vi "Abort.vi"() -> ()   [LabVIEW 2024]
uses:
  states.ctl
  <vilib>/regexp/Match Regular Expression.xnode
panel:
  out "RunningVIs":string[][](table)
  in  "Exit":bool
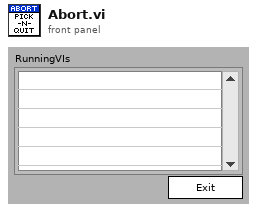
[diagram p1: front panel]
types:
  T1 = typedef "states.ctl" = enum16{"Idle", "Data: Initialize", "Data: get contexts", "Data: get running VIs", "Data: count running", "Macro: Initialize", "Macro: get VIs", "Script: abort VI", "Exit"}
  T2 = enum32{"Bad", "Idle", "Run top level", "Running"}
  T3 = typedef "LVPoint32TypeDef.ctl" = cluster{"Horizontal":i32, "Vertical":i32}
  T4 = typedef "LVRowAndColumnTypeDef.ctl" = cluster{"Row":i32, "Column":i32}
  T5 = cluster{"Core":cluster{"Current VI Reference":refnum<vi>, "Close Panel on Exit?":bool}, "RunningVIRefs":refnum<vi>[], "RunningVINames":string[], "ContextRefs":refnum<vi>[], "SelectedRow":i32}
  T6 = cluster{"Current VI Reference":refnum<vi>, "Close Panel on Exit?":bool}
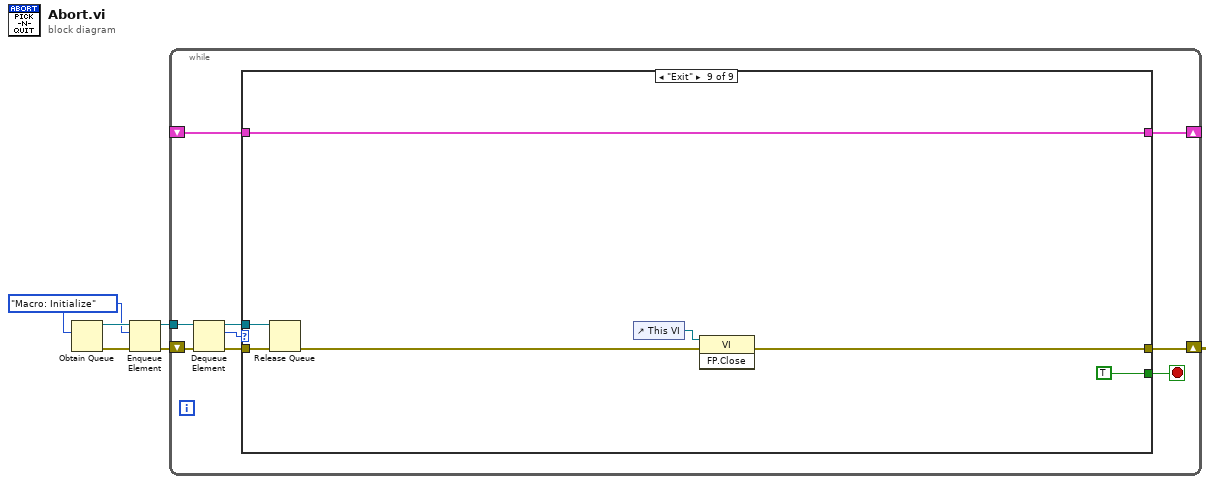
[diagram p0: block diagram]
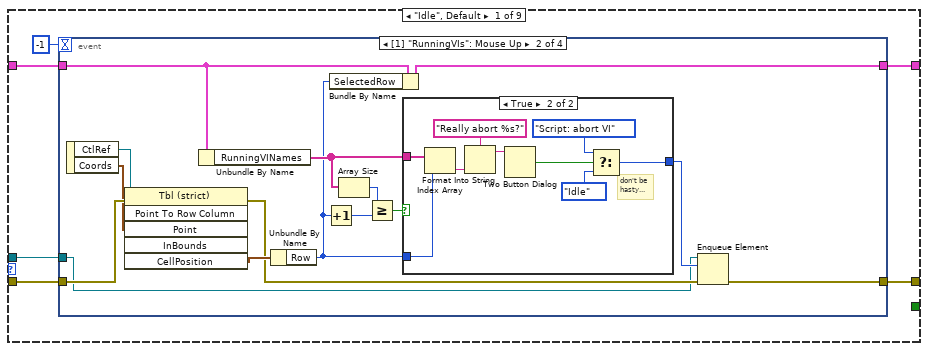
[diagram p2: hidden frame]
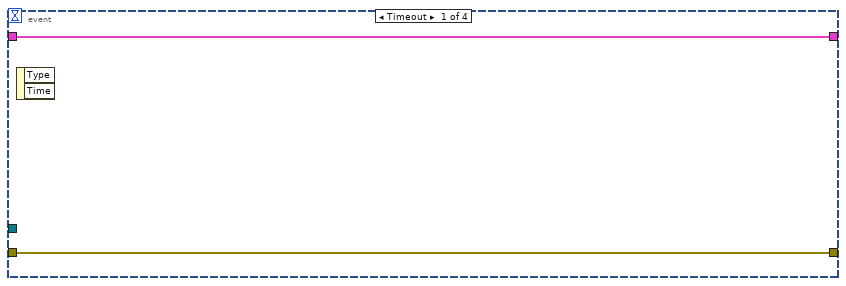
[diagram p3: hidden frame]
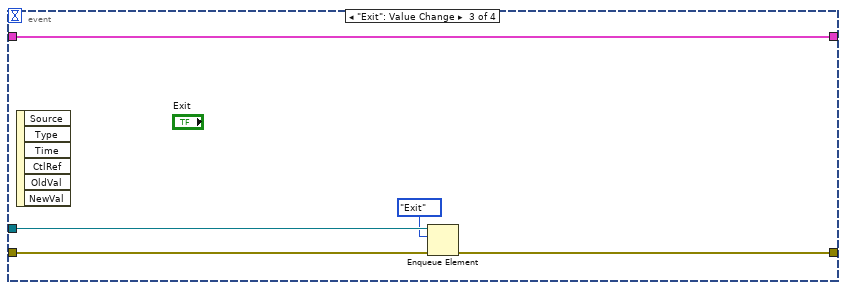
[diagram p5: hidden frame]
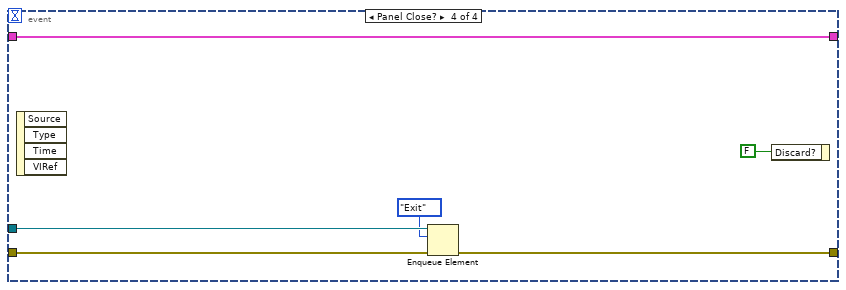
[diagram p6: hidden frame]
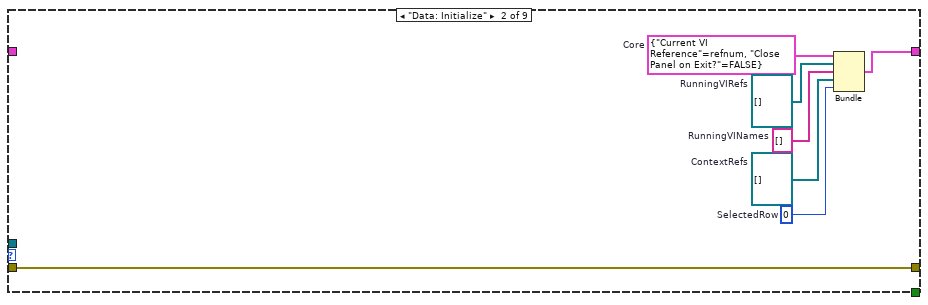
[diagram p7: hidden frame]
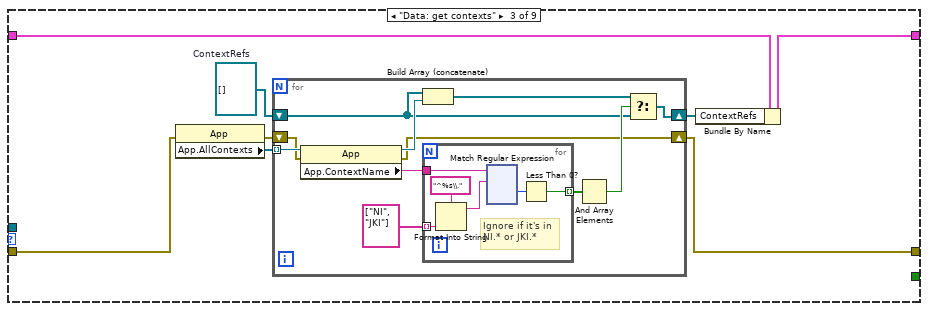
[diagram p8: hidden frame]
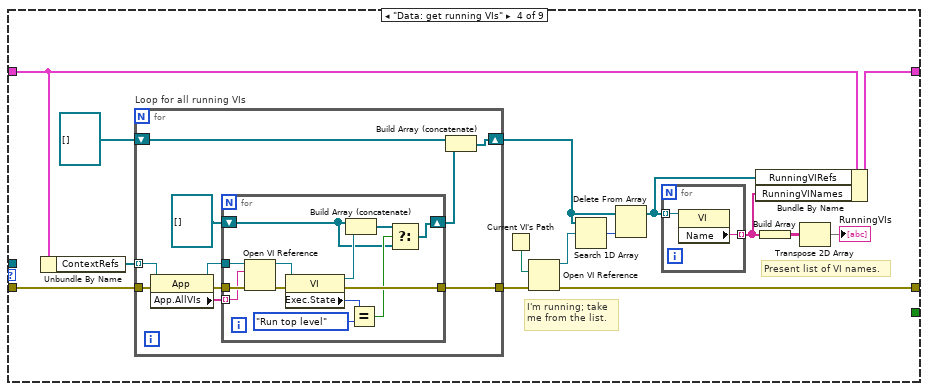
[diagram p9: hidden frame]
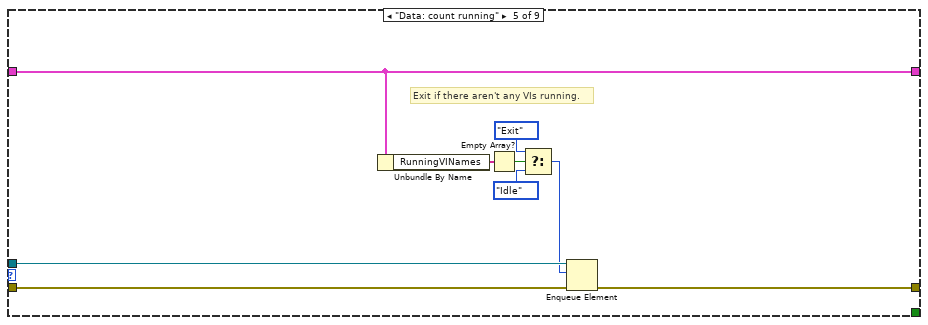
[diagram p10: hidden frame]
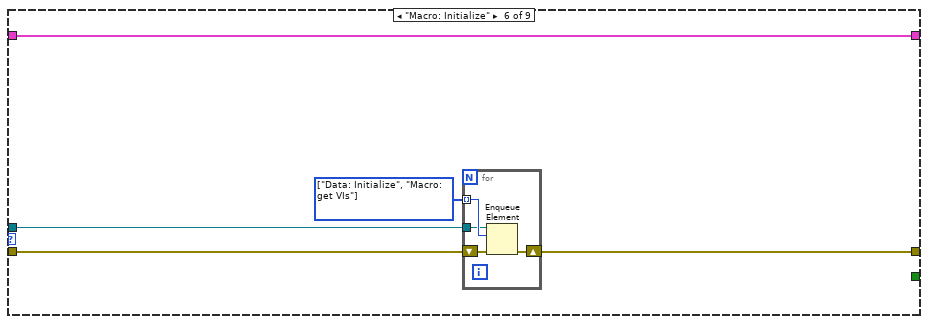
[diagram p11: hidden frame]
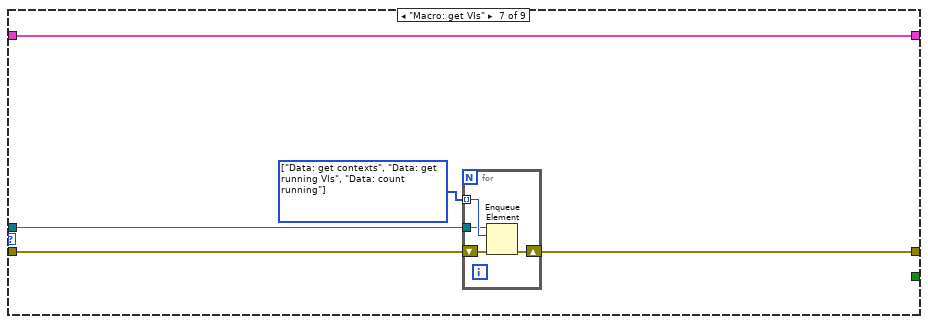
[diagram p12: hidden frame]
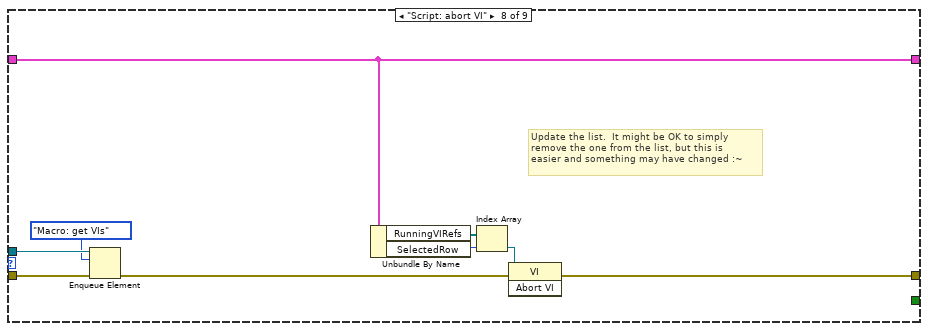
[diagram p13: hidden frame]
diagram:
  w3 = states."Macro: Initialize" ("States")
  n1 = Obtain Queue(element data type=w3) -> (queue out=w4:refnum<queue>, error out=w5:errorcluster)  [unwired: 4 in, 1 out]
  n2 = Enqueue Element(queue=w4, element=w3, error in (no error)=w5) -> (queue out=w1:refnum<queue>, error out=w2:errorcluster)  [unwired: 1 in, 1 out]
  n3 = while {
    tunnel: w1 -> [w13]
    shift-right: [w11] -> _
    shift-left: w2 -> [w14]
    shift-right: [w9] -> _
    shift-left: _ -> [w8]
    stop <- w6 stop-if-true
    n4 = Dequeue Element(queue=w13, error in (no error)=w14) -> (queue out=w7:refnum<queue>, element=w12:T1, error out=w10:errorcluster)  [unwired: 1 in, 1 out]
    n5 = case shown="\"Exit\"" w12 {
      tunnel: [w20 w60 w68 w208 w250 w259 w267 w279 w284] -> w11
      tunnel: w10 -> [w19 w60 w69 w211 w252 w260 w268 w280 w288]
      tunnel: [w18 w59 w66 w209 w253 w256 w265 w278 w285] -> w9
      tunnel: w8 -> [w17 _ w67 w210 w253 w256 w265 w278 w285]
      tunnel: w7 -> [w15 _ _ _ w251 w257 w266 w275 w287]
      tunnel: [_ _ _ _ _ _ _ _ TRUE] -> w6
      frame "Idle", Default {
        n6 = event shown="[1] \"RunningVIs\": Mouse Up" {
          selector: _ -> [_ _ _ _]
          dyn-events: _ -> [_ _ _ _]
          timeout: -1 -> [_ _ _ _]
          tunnel: [w22 w25 w49 w55] -> w20
          tunnel: w19 -> [w22 w31 w51 w57]
          tunnel: [w21 w27 w47 w52] -> w18
          tunnel: w17 -> [w21 w32 w47 w52]
          tunnel: w15 -> [_ w23 w50 w56]
          event Timeout {
            n7 = event-data() -> ()  [unwired: 1 in, 2 out]
          }
          event "RunningVIs": Mouse Up {
            n8 = event-data() -> ("CtlRef"=w29:refnum<vi>, "Coords"=w30:T3)  [unwired: 1 in]
            n9 = invoke class="Tbl (strict)" method="Point To Row Column"(reference=w29, error in=w31, "Point"=w30) -> (error out=w28:errorcluster, "CellPosition"=w33:T4)  [unwired: 3 in, 4 out]
            n10 = Unbundle By Name(w32) -> ("RunningVINames"=w34:string[])
            n11 = Unbundle By Name(w33) -> ("Row"=w26:i32)
            n12 = Increment(x=w26) -> (x+1=w36:i32)
            n13 = Bundle By Name(cluster=w32, "SelectedRow"=w26) -> (w27:T5)
            n14 = Array Size(array=w34) -> (size(s)=w35:i32)
            n15 = Greater Or Equal?(x=w35, y=w36) -> (x >= y?=w37:bool)
            n16 = case shown="True" w37 {
              tunnel: [_ w46] -> w24
              tunnel: w34 -> [_ w41]
              tunnel: w26 -> [_ w38]
              frame False {
                # "don't respond if an empty\nrow was selected"
              }
              frame True {
                # "don't be\nhasty..."
                n17 = Index Array(array=w41, index=w38) -> (element=w42:string)
                n18 = Format Into String(format string="Really abort %s?", w42) -> (resulting string=w43:string)  [unwired: 2 in, 1 out]
                n19 = Two Button Dialog(message=w43) -> (T button?=w45:bool)  [unwired: 2 out]
                n20 = Select(t=states."Script: abort VI" ("States"), s=w45, f=states."Idle" ("States")) -> (s? t:f=w46:T1)
              }
            }
            n21 = Enqueue Element(queue=w23, element=w24, error in (no error)=w28) -> (error out=w25:errorcluster)  [unwired: 1 in, 2 out]
          }
          event "Exit": Value Change {
            n22 = event-data() -> ()  [unwired: 1 in, 6 out]
            n23 = Enqueue Element(queue=w50, element=states."Exit", error in (no error)=w51) -> (error out=w49:errorcluster)  [unwired: 1 in, 2 out]
          }
          event Panel Close? {
            n24 = event-data() -> ()  [unwired: 1 in, 4 out]
            n25 = Enqueue Element(queue=w56, element=states."Exit", error in (no error)=w57) -> (error out=w55:errorcluster)  [unwired: 1 in, 2 out]
            n26 = event-data("Discard?"=FALSE) -> ()  [unwired: 1 in, 1 out]
          }
        }
      }
      frame "Data: Initialize" {
        w58 = 0  # SelectedRow
        w64 = refnum<vi>[] []  # ContextRefs
        w63 = string[] []  # RunningVINames
        w62 = refnum<vi>[] []  # RunningVIRefs
        w61 = T6 {"Current VI Reference"=refnum, "Close Panel on Exit?"=FALSE}  # Core
        n27 = Bundle("Core"=w61, "RunningVIRefs"=w62, "RunningVINames"=w63, "ContextRefs"=w64, "SelectedRow"=w58) -> (w59:T5)  [unwired: 1 out]
      }
      frame "Data: get contexts" {
        w72 = refnum<vi>[] []  # ContextRefs
        n28 = property class="App"(error in=w69) -> (error out=w71:errorcluster, "App.AllContexts"=w70:refnum<vi>[])  [unwired: 1 in, 1 out]
        n29 = for {
          tunnel: w70 -> [w83] mode=indexing
          shift-right: [w74] -> w65
          shift-left: w72 -> [w75]
          shift-right: [w73] -> w68
          shift-left: w71 -> [w80]
          n30 = property class="App"(reference=w83, error in=w80) -> (reference out=w77:refnum<vi>, error out=w73:errorcluster, "App.ContextName"=w81:string)
          n31 = Build Array (concatenate)(w75, w77) -> (w76:refnum<vi>[])
          n32 = for {
            tunnel: string[] ["NI", "JKI"] -> [w87] mode=indexing
            tunnel: w81 -> [w89]
            tunnel: [w84] -> w79 mode=indexing
            # "Ignore if it's in\nNI.* or JKI.*"
            n33 = Format Into String(format string="^%s\\.", w87) -> (resulting string=w86:string)  [unwired: 2 in, 1 out]
            n34 = xnode "Match Regular Expression"("input string"=w89, "regular expression"=w86) -> ("offset past match"=w85:i32)  [unwired: 2 in, 6 out]
            n35 = Less Than 0?(x=w85) -> (x < 0?=w84:bool)
          }
          n36 = And Array Elements(Boolean array=w79) -> (logical AND=w78:bool)
          n37 = Select(t=w76, s=w78, f=w75) -> (s? t:f=w74:refnum<vi>[])
        }
        n38 = Bundle By Name(cluster=w67, "ContextRefs"=w65) -> (w66:T5)
      }
      frame "Data: get running VIs" {
        # "Present list of VI names."
        # "I'm running; take\nme from the list."
        n39 = Unbundle By Name(w210) -> ("ContextRefs"=w213:refnum<vi>[])
        n40 = for "Loop for all running VIs" {
          tunnel: w211 -> [w227]
          tunnel: [w225] -> w218
          tunnel: w213 -> [w226] mode=indexing
          shift-right: [w232] -> w219
          shift-left: refnum<vi>[] [] ("VIRefs") -> [w233]
          n41 = property class="App"(reference=w226, error in=w227) -> (reference out=w230:refnum<vi>, error out=w231:errorcluster, "App.AllVIs"=w229:string[])
          n42 = for {
            tunnel: w231 -> [w246]
            tunnel: w230 -> [w244]
            tunnel: w229 -> [w245] mode=indexing
            shift-right: [w234] -> w224
            shift-left: refnum<vi>[] [] ("RunningVIRefs 2") -> [w235]
            tunnel: [w238] -> w225
            n43 = Open VI Reference(application reference (local)=w244, vi path=w245, error in (no error)=w246) -> (vi reference=w243:refnum<vi>, error out=w242:errorcluster)  [unwired: 3 out]
            n44 = property class="VI"(reference=w243, error in=w242) -> (reference out=w239:refnum<vi>, error out=w238:errorcluster, "Exec.State"=w241:T2)
            n45 = Build Array (concatenate)(w235, w239) -> (w236:refnum<vi>[])
            n46 = Equal?(x=w241, y=T2."Run top level" ("Execution:State")) -> (x = y?=w237:bool)
            n47 = Select(t=w236, s=w237, f=w235) -> (s? t:f=w234:refnum<vi>[])
          }
          n48 = Build Array (concatenate)(w233, w224) -> (w232:refnum<vi>[])
        }
        n49 = Current VI's Path() -> (path=w217:path)
        n50 = Open VI Reference(vi path=w217, error in (no error)=w218) -> (vi reference=w216:refnum<vi>, error out=w208:errorcluster)  [unwired: 4 out]
        n51 = Search 1D Array(1D array=w219, element=w216) -> (index of element=w215:i32)  [unwired: 1 out]
        n52 = Delete From Array(array=w219, index=w215) -> (array with subset deleted=w220:refnum<vi>[])  [unwired: 1 in, 1 out]
        n53 = for {
          tunnel: w220 -> [w223] mode=indexing
          tunnel: [w222] -> w221 mode=indexing
          n54 = property class="VI"(reference=w223) -> ("Name"=w222:string)  [unwired: 1 in, 2 out]
        }
        n55 = Bundle By Name(cluster=w210, "RunningVIRefs"=w220, "RunningVINames"=w221) -> (w209:T5)
        n56 = Build Array(w221) -> (w212:string[][])
        n57 = Transpose 2D Array(2D array=w212) -> (transposed array=→"RunningVIs":string[][])
      }
      frame "Data: count running" {
        # "Exit if there aren't any VIs running."
        n58 = Unbundle By Name(w253) -> ("RunningVINames"=w254:string[])
        n59 = Empty Array?(array=w254) -> (empty?=w255:bool)
        n60 = Select(t=states."Exit" ("States"), s=w255, f=states."Idle" ("States")) -> (s? t:f=w247:T1)
        n61 = Enqueue Element(queue=w251, element=w247, error in (no error)=w252) -> (error out=w250:errorcluster)  [unwired: 1 in, 2 out]
      }
      frame "Macro: Initialize" {
        w258 = T1[] [enum."Data: Initialize", enum."Macro: get VIs"] items=["Idle", "Data: Initialize", "Data: get contexts", "Data: get running VIs", "Data: count running", "Macro: Initialize", "Macro: get VIs", "Script: abort VI", "Exit"]
        n62 = for {
          shift-right: [w263] -> w259
          shift-left: w260 -> [w264]
          tunnel: w258 -> [w262] mode=indexing
          tunnel: w257 -> [w261]
          n63 = Enqueue Element(queue=w261, element=w262, error in (no error)=w264) -> (error out=w263:errorcluster)  [unwired: 1 in, 2 out]
        }
      }
      frame "Macro: get VIs" {
        w269 = T1[] [enum."Data: get contexts", enum."Data: get running VIs", enum."Data: count running"] items=["Idle", "Data: Initialize", "Data: get contexts", "Data: get running VIs", "Data: count running", "Macro: Initialize", "Macro: get VIs", "Script: abort VI", "Exit"]
        n64 = for {
          shift-right: [w272] -> w267
          shift-left: w268 -> [w273]
          tunnel: w269 -> [w271] mode=indexing
          tunnel: w266 -> [w270]
          n65 = Enqueue Element(queue=w270, element=w271, error in (no error)=w273) -> (error out=w272:errorcluster)  [unwired: 1 in, 2 out]
        }
      }
      frame "Script: abort VI" {
        # "Update the list.  It might be OK to simply\nremove the one from the list, but this is\neasier and something may have changed :~"
        n66 = Enqueue Element(queue=w275, element=states."Macro: get VIs", error in (no error)=w280) -> (error out=w276:errorcluster)  [unwired: 1 in, 2 out]
        n67 = Unbundle By Name(w278) -> ("RunningVIRefs"=w281:refnum<vi>[], "SelectedRow"=w277:i32)
        n68 = Index Array(array=w281, index=w277) -> (element=w282:refnum<vi>)
        n69 = invoke class="VI" method="Abort VI"(reference=w282, error in=w276) -> (error out=w279:errorcluster)  [unwired: 1 in, 2 out]
      }
      frame "Exit" {
        n70 = Release Queue(queue=w287, error in (no error)=w288) -> (error out=w286:errorcluster)  [unwired: 1 in, 2 out]
        n71 = control-ref of="This VI"() -> (w283:refnum<vi>)
        n72 = invoke class="VI" method="FP.Close"(reference=w283, error in=w286) -> (error out=w284:errorcluster)  [unwired: 1 in, 2 out]
      }
    }
  }
